vi "control state select tree.vi"() -> (2 "Control_State":T1)   [LabVIEW 2020]
uses:
  LED_Control_States.ctl
  <vilib>/Rock Robotics/WPI/DriverStation/WPI_DriverStationRobotMode2.ctl
  Robot Global Data.vi
  Globals/Climber_Globals.vi
  Globals/Flywheel_Globals.vi
  Globals/Turret_Globals.vi
  Globals/Cowl_Globals.vi
  Globals/Sensor_Values.vi
  Globals/Autonomous_Globals.vi
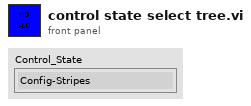
[diagram p1: front panel]
types:
  T1 = typedef "LED_Control_States.ctl" = enum16{"Config-Stripes", "swapperlines", "Rand", "Solid", "Flash-S", "Gradyent", "Move-Stripes", "Org-Rand", "Move-Point-Tail", "Flames", "Fade", "Alt-Colors"}
  T2 = typedef "WPI_DriverStationRobotMode2.ctl" = enum16{"Autonomous Disabled", "Autonomous Enabled", "Teleop Disabled", "Teleop Enabled", "Disconnected", "Finish", "Test Disabled", "Test Enabled", "Emergency Stopped"}
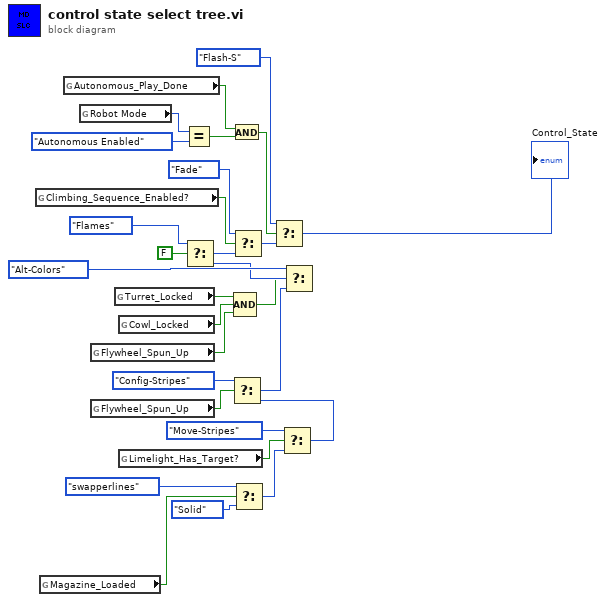
[diagram p0: block diagram]
diagram:
  n1 = global read "Climber_Globals.vi" "Climbing_Sequence_Enabled?"() -> (w14:bool)
  n2 = global read "Sensor_Values.vi" "Magazine_Loaded"() -> (w7:bool)
  n3 = global read "Autonomous_Globals.vi" "Autonomous_Play_Done"() -> (w5:bool)
  n4 = global read "Robot Global Data.vi" "Robot Mode"() -> (w16:T2)
  n5 = global read "Flywheel_Globals.vi" "Flywheel_Spun_Up"() -> (w1:bool)
  n6 = global read "Flywheel_Globals.vi" "Flywheel_Spun_Up"() -> (w11:bool)
  n7 = global read "Turret_Globals.vi" "Turret_Locked"() -> (w3:bool)
  n8 = global read "Cowl_Globals.vi" "Cowl_Locked"() -> (w2:bool)
  n9 = global read "Sensor_Values.vi" "Limelight_Has_Target?"() -> (w8:bool)
  n10 = Equal?(x=w16, y=WPI_DriverStationRobotMode2."Autonomous Enabled") -> (x = y?=w6:bool)
  n11 = And(x=w5, y=w6) -> (x .and. y?=w4:bool)
  n12 = Compound Arithmetic op=AND(w3, w2, w1) -> (w12:bool)
  n13 = Select(t=LED_Control_States."swapperlines" ("Control_State"), s=w7, f=LED_Control_States."Solid" ("Control_State")) -> (s? t:f=w10:T1)
  n14 = Select(t=LED_Control_States."Move-Stripes" ("Control_State"), s=w8, f=w10) -> (s? t:f=w9:T1)
  n15 = Select(t=LED_Control_States."Config-Stripes" ("Control_State"), s=w11, f=w9) -> (s? t:f=w17:T1)
  n16 = Select(t=LED_Control_States."Alt-Colors" ("Control_State"), s=w12, f=w17) -> (s? t:f=w20:T1)
  n17 = Select(t=LED_Control_States."Flames" ("Control_State"), s=FALSE, f=w20) -> (s? t:f=w19:T1)
  n18 = Select(t=LED_Control_States."Fade" ("Control_State"), s=w14, f=w19) -> (s? t:f=w18:T1)
  n19 = Select(t=LED_Control_States."Flash-S" ("Control_State"), s=w4, f=w18) -> (s? t:f=→"Control_State":T1)
